vi "Start position (SILAR).vi"(8 "Error In":errorcluster, 11 "Arduino Resource In":T1={"VISA resource"="", "Board Type"=enum."Uno", "Connection Type"=enum."USB / Serial", "Bytes Per Packet (15)"=15}) -> (0 "Error Out":errorcluster, 3 "Arduino Resource Out":T1={"VISA resource"="", "Board Type"=enum."Uno", "Connection Type"=enum."USB / Serial", "Bytes Per Packet (15)"=15})   [LabVIEW 2016]
uses:
  <vilib>/LabVIEW Interface for Arduino/Type Defs/Arduino Resource.ctl
  <vilib>/LabVIEW Interface for Arduino/Type Defs/Board Type.ctl
  <vilib>/LabVIEW Interface for Arduino/LabVIEW Interface for Arduino.lvlib
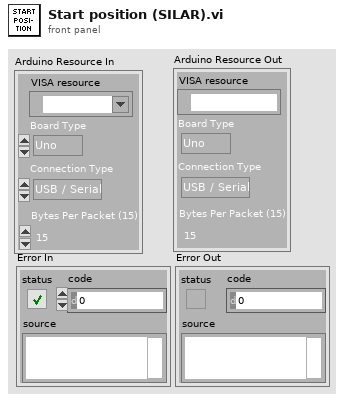
[diagram p1: front panel]
types:
  T1 = typedef "LabVIEW Interface for Arduino.lvlib/Arduino Resource.ctl" = cluster{"VISA resource":refnum<visa-resource-name>, "Board Type":T2, "Connection Type":enum8{"USB / Serial"}, "Bytes Per Packet (15)":u8}
  T2 = typedef "LabVIEW Interface for Arduino.lvlib/Board Type.ctl" = enum16{"Uno", "Dimuelanove w/Atmega 328", "Mega 2560"}
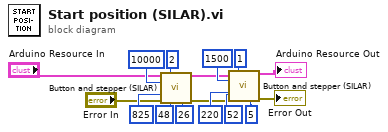
[diagram p0: block diagram]
diagram:
  n1 = call "Button and stepper (SILAR).vi"("Arduino Resource In"="Arduino Resource In", "Шаговый двигатель №"=u8 2 ("Stepper #"), "Кол-во шагов"=i16 10000 ("# of Steps to Move"), "Скорость двигателя"=i16 825 ("Set Speed (Steps per Second)"), "Error In"="Error In", "Контакт концевика"=u8 48 ("Digital I/O Pin (0)"), "ENABLE контакт"=u8 26 ("ENABLE Pin")) -> ("Arduino Resource Out"=w6:T1, "Error Out"=w5:errorcluster)  [unwired: 7 in]
  n2 = call "Button and stepper (SILAR).vi"("Arduino Resource In"=w6, "Шаговый двигатель №"=u8 1 ("Stepper #"), "Кол-во шагов"=i16 1500 ("# of Steps to Move"), "Скорость двигателя"=i16 220 ("Set Speed (Steps per Second)"), "Error In"=w5, "Контакт концевика"=u8 52 ("Digital I/O Pin (0)"), "ENABLE контакт"=u8 5 ("ENABLE Pin")) -> ("Arduino Resource Out"=→"Arduino Resource Out":T1, "Error Out"=→"Error Out":errorcluster)  [unwired: 7 in]
